vi "SubVI_Example_StartLive.vi"(8 "Error":errorcluster caption="Error In", 11 ".NET (Reference)":refnum<k24>) -> (0 "Error":errorcluster caption="Error Out")   [LabVIEW 2010]
uses:
  C:/Program Files (x86)/National Instruments/LabVIEW 2016/instr.lib/IDS/ueye.NET/uEyeDotNet.dll
  Program Files (x86)/National Instruments/LabVIEW 2016/instr.lib/IDS/ueye.NET/uEyeDotNet.dll
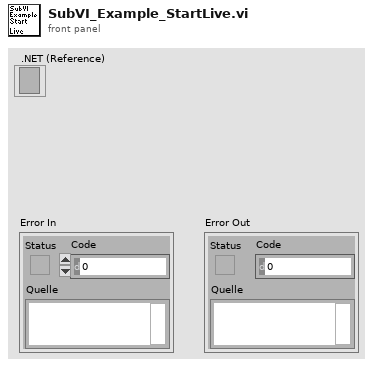
[diagram p1: front panel]
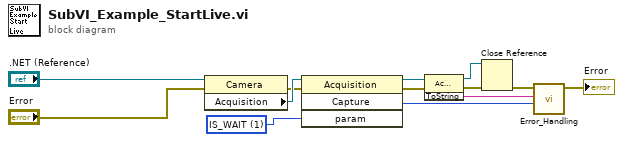
[diagram p0: block diagram]
diagram:
  w7 = 1 items=["IS_DONT_WAIT", "IS_WAIT"] ("Wait")
  n1 = property class="Camera"(reference=".NET (Reference)", error in="Error") -> (error out=w12:errorcluster, "Acquisition"=w13:refnum<k24>)  [unwired: 1 out]
  n2 = invoke class="Acquisition" method="Capture"(reference=w13, error in=w12, "param"=w7) -> (reference out=w9:refnum<k24>, error out=w10:errorcluster, "Capture"=w8:i32)  [unwired: 1 in, 1 out]
  n3 = invoke class="Acquisition" method="ToString"(reference=w9, error in=w10) -> (reference out=w1:refnum<k24>, error out=w3:errorcluster, "ToString"=w11:string)  [unwired: 1 in]
  n4 = Close Reference(reference=w1, error in (no error)=w3) -> (error out=w2:errorcluster)
  n5 = call "Error_Handling.vi"("Error Code"=w8, "Error String"=w11, "Error In"=w2) -> ("Error Out"=→"Error":errorcluster)  [unwired: 8 in]
